vi "ReadUnicodeText.vi"(8 "txtIn":string) -> (1 "result string":string)   [LabVIEW 2018]
uses:
  kernel32.dll
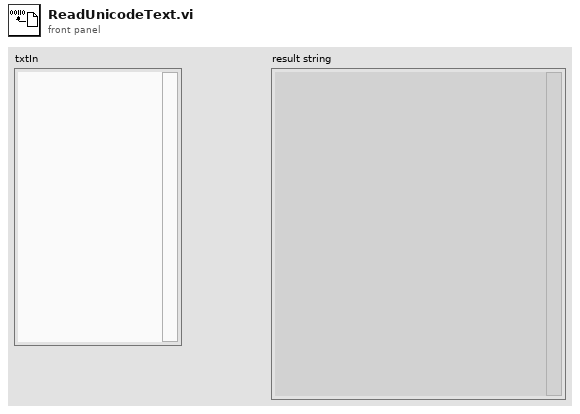
[diagram p1: front panel]
types:
  T1 = enum16{"big-endian, network order", "native, host order", "little-endian"}
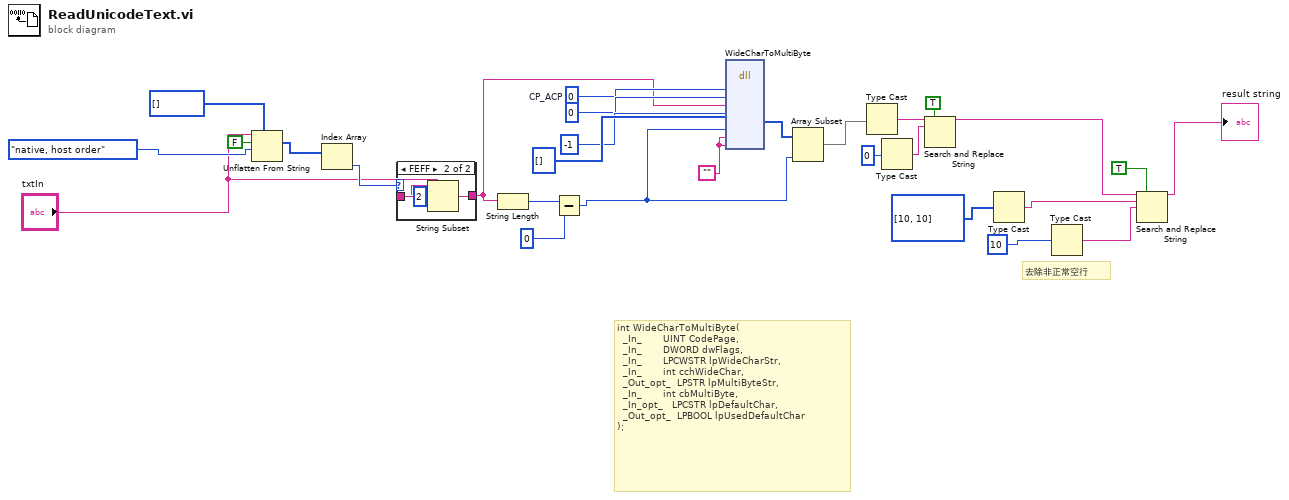
[diagram p0: block diagram]
diagram:
  w20 = u32 0  # CP_ACP
  w23 = ""
  # "去除非正常空行"
  # "int WideCharToMultiByte(\n  _In_       UINT CodePage,\n  _In_       DWORD dwFlags,\n  _In_       LPCWSTR lpWideCharStr,\n  _In_       int cchWideChar,\n  _Out_opt_  LPSTR lpMultiByteStr,\n  _In_       int cbMultiByte,\n  _In_opt_   LPCSTR lpDefaultChar,\n  _Out_opt_  LPBOOL lpUsedDefaultChar\n);"
  n1 = Unflatten From String(type=u16[] [] ("lpWideCharStr"), binary string="txtIn", data includes array or string size? (T)=FALSE ("数据中包含数组或字符串大小？(T)"), byte order (0:big-endian, network order)=T1."native, host order" ("字节顺序(0:big-endian, network order)")) -> (value=w8:u16[])  [unwired: 1 in, 2 out]
  n2 = Index Array(array=w8) -> (element=w10:u16)  [unwired: 1 in]
  n3 = case shown="FEFF" w10 {
    tunnel: "txtIn" -> [w29 w31]
    tunnel: [w29 w30] -> w6
    frame Default {
    }
    frame 65279 {
      n4 = String Subset(string=w31, offset (0)=2 ("偏移量(0)")) -> (substring=w30:string)  [unwired: 1 in]
    }
  }
  n5 = String Length(string=w6) -> (length=w2:i32)
  n6 = Subtract(x=w2, y=0) -> (x-y=w1:i32)
  n7 = dll-call lib="kernel32.dll" fn="WideCharToMultiByte"("CodePage"=w20, "dwFlags"=0, "lpWideCharStr"=w6, "cchWideChar"=-1, "lpMultiByteStr"=u8[] [], "cchMultiByte"=w1, "lpDefaultChar"=w23, "pfUsedDefaultChar"=w23) -> ("lpMultiByteStr"=w4:u8[])  [unwired: 11 in, 2 out]
  n8 = Array Subset(array=w4, length=w1) -> (w3:u8[])  [unwired: 1 in]
  n9 = Type Cast(x=w3) -> (*(type *) &x=w26:string)  [unwired: 1 in]
  n10 = Type Cast(x=u8 0 ("元素")) -> (*(type *) &x=w24:string)  [unwired: 1 in]
  n11 = Search and Replace String(replace all?=TRUE ("替换全部？(F)"), input string=w26, search string=w24) -> (result string=w18:string)  [unwired: 5 in, 3 out]
  n12 = Type Cast(x=u8[] [10, 10]) -> (*(type *) &x=w15:string)  [unwired: 1 in]
  n13 = Type Cast(x=u8 10 ("元素")) -> (*(type *) &x=w14:string)  [unwired: 1 in]
  n14 = Search and Replace String(replace all?=TRUE ("替换全部？(F)"), input string=w18, search string=w15, replace string=w14) -> (result string=→"result string":string)  [unwired: 4 in, 3 out]
